vi "Heater.vi"() -> ()   [LabVIEW 2012]
panel:
  out "Heater On/Off":bool
  in  "Allow Heater On?":bool
  in  "RTD1 Setpoint":dbl=165.0
  in  "SettlingFactor":i32
  in  "Resolution":i32=12
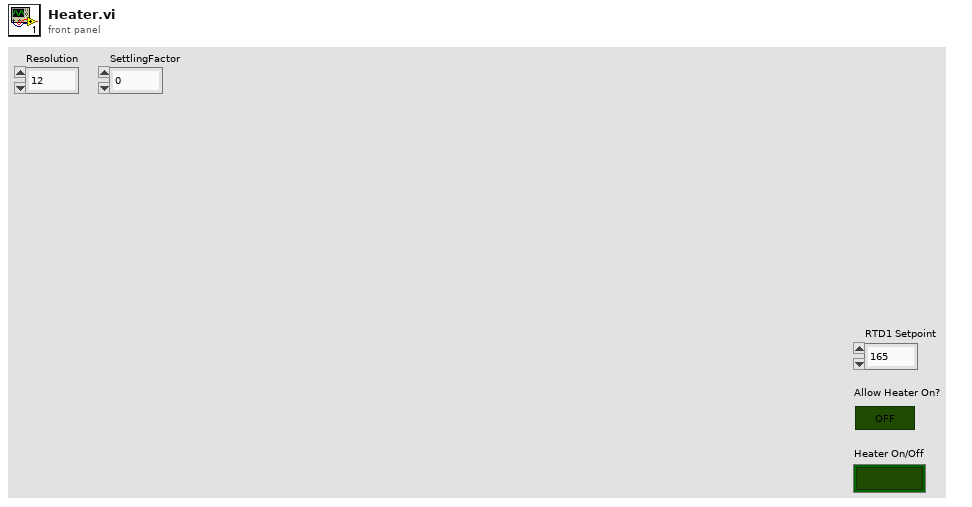
[diagram p1: front panel]
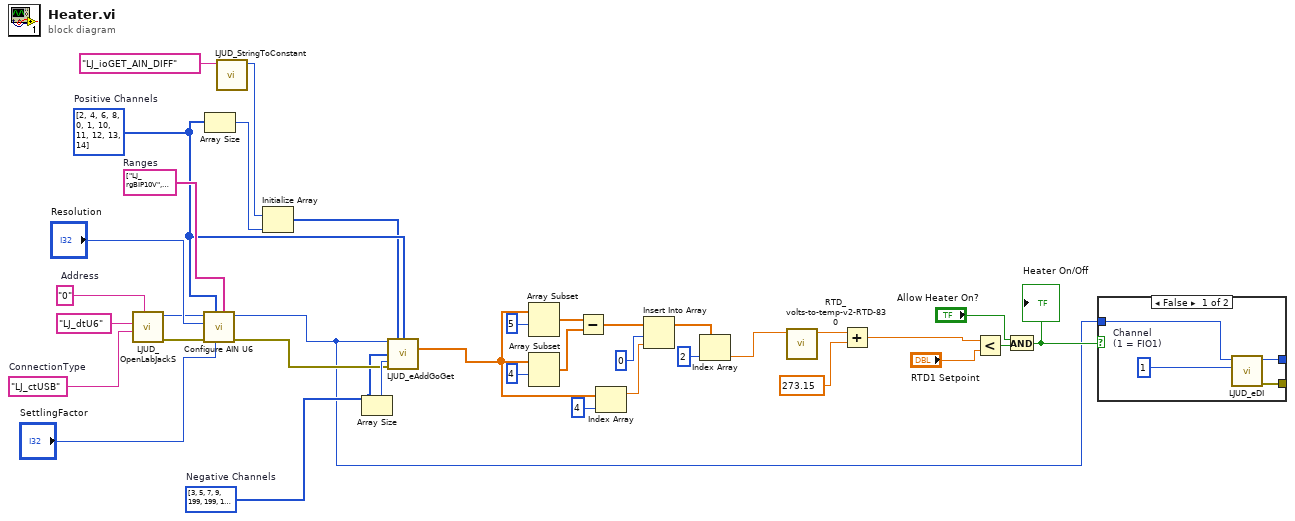
[diagram p0: block diagram]
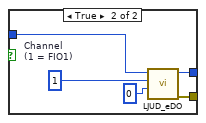
[diagram p2: hidden frame]
diagram:
  w21 = i32[] [3, 5, 7, 9, 199, 199, 199, 199, 199, 199, 199]  # Negative Channels
  w35 = string[] ["LJ_rgBIP10V", "LJ_rgBIP10V", "LJ_rgBIP10V", "LJ_rgBIP10V", "LJ_rgBIP1V", "LJ_rgBIP1V", "LJ_rgBIP1V", "LJ_rgBIP1V", "LJ_rgBIP1V", "LJ_rgBIP1V", "LJ_rgBIP10V"]  # Ranges
  w24 = i32[] [2, 4, 6, 8, 0, 1, 10, 11, 12, 13, 14]  # Positive Channels
  w29 = "0"  # Address
  w31 = "LJ_ctUSB"  # ConnectionType
  n1 = call <vilib>:"LJUD_OpenLabJackS.vi"("Address"=w29, "ConnectionType"=w31, "DeviceType"="LJ_dtU6") -> ("error out"=w33:errorcluster, "Handle"=w32:i32)  [unwired: 6 in, 1 out]
  n2 = call <vilib>:"Configure AIN U6.vi"("Ranges"=w35, "SettlingFactor"="SettlingFactor", "Positive Channels"=w24, "error in"=w33, "Resolution"="Resolution", "Handle In"=w32) -> ("error out"=w22:errorcluster, "Handle Out"=w7:i32)  [unwired: 4 in]
  n3 = Array Size(array=w24) -> (size(s)=w36:i32)
  n4 = call <vilib>:"LJUD_StringToConstant.vi"("String"="LJ_ioGET_AIN_DIFF" ("IOType")) -> ("Constant Number"=w26:i32)  [unwired: 9 in, 1 out]
  n5 = Initialize Array(w26, w36) -> (w23:i32[])
  n6 = Array Size(array=w21) -> (size(s)=w25:i32)
  n7 = call <vilib>:"LJUD_eAddGoGet.vi"("Handle In"=w7, "aIOTypes"=w23, "aChannels"=w24, "ax1s"=w21, "NumRequests"=w25, "error in"=w22) -> ("Values Read"=w12:dbl[])  [unwired: 4 in, 5 out]
  n8 = Array Subset(array=w12, index=5 ("Index")) -> (w17:dbl[])  [unwired: 1 in]
  n9 = Array Subset(array=w12, index=4 ("Index")) -> (w19:dbl[])  [unwired: 1 in]
  n10 = Subtract(x=w17, y=w19) -> (x-y=w16:dbl[])
  n11 = Index Array(array=w12, index=4) -> (element=w13:dbl)
  n12 = Insert Into Array(array=w16, index=0 ("Index"), new element=w13) -> (w5:dbl[])
  n13 = Index Array(array=w5, index=2) -> (element=w2:dbl)
  n14 = call "RTD_volts-to-temp-v2-RTD-830.vi"("RTD Volts"=w2) -> ("Temp"=w3:dbl)  [unwired: 10 in]
  n15 = Add(x=w3, y=273.15) -> (x+y=w1:dbl)
  n16 = Less?(x=w1, y="RTD1 Setpoint") -> (x < y?=w9:bool)
  n17 = And(x="Allow Heater On?", y=w9) -> (x .and. y?=w11:bool)
  "Heater On/Off" <- w11
  n18 = case shown="False" w11 {
    tunnel: [w39 w43] -> _
    tunnel: [w38 w42] -> _
    tunnel: w7 -> [w37 w41]
    frame False {
      w40 = 1  # Channel (1 = FIO1)
      n19 = call <vilib>:"LJUD_eDI.vi"("Channel"=w40, "Handle In"=w37) -> ("error out"=w39:errorcluster, "Handle Out"=w38:i32)  [unwired: 7 in, 1 out]
    }
    frame True {
      w44 = 1  # Channel (1 = FIO1)
      n20 = call <vilib>:"LJUD_eDO.vi"("State"=0, "Channel"=w44, "Handle In"=w41) -> ("error out"=w43:errorcluster, "Handle Out"=w42:i32)  [unwired: 7 in]
    }
  }
